vi "Get Cluster Element Type.vi"(8 "error in (no error)":errorcluster, 10 "Element Name":string, 11 "Cluster in":variant) -> (0 "error out":errorcluster, 2 "Type":variant, 3 "Cluster out":variant)   [LabVIEW 2015, in "Scripting.lvlib"]
doc: "<B>Type</B> is the type of the element with name <B>Element Name</B> in <B>Cluster in</B>"
uses:
  Scripting.lvlib
  <vilib>/Utility/Data Type/NI_Data Type.lvlib
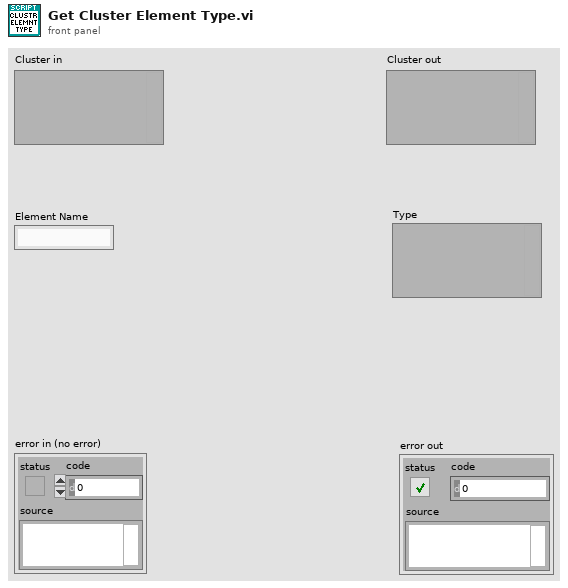
[diagram p1: front panel]
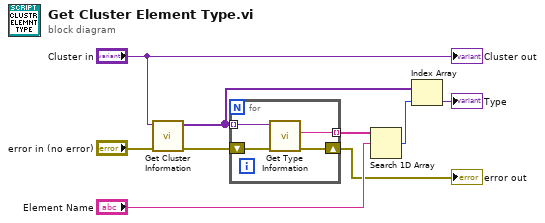
[diagram p0: block diagram]
diagram:
  n1 = call <vilib>:"Get Cluster Information.vi"("error in (no error)"="error in (no error)", "Variant"="Cluster in") -> ("error out"=w3:errorcluster, "Cluster Elements"=w7:variant[])  [unwired: 8 in]
  n2 = for {
    tunnel: w7 -> [w13] mode=indexing
    tunnel: [w12] -> w8 mode=indexing
    shift-right: [w10] -> w1
    shift-left: w3 -> [w11]
    n3 = call <vilib>:"Get Type Information.vi"("error in (no error)"=w11, "Variant"=w13) -> ("error out"=w10:errorcluster, "Name"=w12:string)  [unwired: 5 in, 3 out]
  }
  "error out" <- w1
  n4 = Search 1D Array(1D array=w8, element="Element Name") -> (index of element=w9:i32)  [unwired: 1 in]
  n5 = Index Array(array=w7, index=w9) -> (element=→"Type":variant)
  "Cluster out" <- "Cluster in"
